vi "SERIAL_DecodeStreamResponse.vi"(8 "error in":errorcluster, 10 "Buffer":string, 11 "navX DevRef":T1={"SerialPortRef"={"DevStatus"={"status"=FALSE, "code"=0, "source"=""}, "Serial Port Name"=""}, "Board Information"={"WhoAmI (50 | 0x32)"=0, "Board Revision"=0, "Firmware Major Version"=0, "Firmware Minor Version"=0, "NAVX_BOARD_CAPABILITY"={"OMNIMOUNT"=FALSE, "YAW_RESET"=FALSE, "VEL_AND_DISP"=FALSE}, "NAVX_BOARD_YAW_AXIS"={"BOARD_YAW_AXIS_UP"=FALSE, "BOARD_YAW_AXIS"=0}}, "Status"={"Update Rate Hz"=0, "Accelerometer Full-Scale Range"=0, "Gyro Full-Scale Range"=0, "NAVX_OP_STATUS"=0, "NAVX_CAL_STATUS"=0, "NAVX_SELFTEST_STATUS"=0, "NAVX_SENSOR_STATUS"={"MOVING"=FALSE, "YAW_STABLE"=FALSE, "MAG_DISTURBANCE"=FALSE, "ALTITUDE_VALID"=FALSE, "SEALEVEL_PRESS_SET"=FALSE, "FUSED_HEADING_VALID"=FALSE}}, "Offsets"={"Yaw"=0.0, "Quat W"=0.0, "Quat X"=0.0, "Quat Y"=0.0, "Quat Z"=0.0}, "Update Rate (4Hz-60Hz)"=50, "Nav6Mode (YPR)"=enum."YPR", "refnum name"="", "error"={"status"=FALSE, "code"=0, "source"=""}, "Loop VI Refnum"=refnum} {"Status"."NAVX_OP_STATUS" items=["INITIALIZING", "SELFTEST_IN_PROGRESS", "ERROR", "IMU_AUTOCAL_IN_PROGRESS", "NORMAL"]; "Status"."NAVX_CAL_STATUS" items=["IMU_CAL_STATE_MASK"=3, "IMU_CAL_INPROGRESS"=0, "IMU_CAL_ACCUMULATE"=1, "IMU_CAL_COMPLETE"=2, "MAG_CAL_COMPLETE"=4, "BARO_CAL_COMPLETE"=8]}) -> (0 "error out":errorcluster, 2 "Valid":bool, 3 "navX DevRef":T1={"SerialPortRef"={"DevStatus"={"status"=FALSE, "code"=0, "source"=""}, "Serial Port Name"=""}, "Board Information"={"WhoAmI (50 | 0x32)"=0, "Board Revision"=0, "Firmware Major Version"=0, "Firmware Minor Version"=0, "NAVX_BOARD_CAPABILITY"={"OMNIMOUNT"=FALSE, "YAW_RESET"=FALSE, "VEL_AND_DISP"=FALSE}, "NAVX_BOARD_YAW_AXIS"={"BOARD_YAW_AXIS_UP"=FALSE, "BOARD_YAW_AXIS"=0}}, "Status"={"Update Rate Hz"=0, "Accelerometer Full-Scale Range"=0, "Gyro Full-Scale Range"=0, "NAVX_OP_STATUS"=0, "NAVX_CAL_STATUS"=0, "NAVX_SELFTEST_STATUS"=0, "NAVX_SENSOR_STATUS"={"MOVING"=FALSE, "YAW_STABLE"=FALSE, "MAG_DISTURBANCE"=FALSE, "ALTITUDE_VALID"=FALSE, "SEALEVEL_PRESS_SET"=FALSE, "FUSED_HEADING_VALID"=FALSE}}, "Offsets"={"Yaw"=0.0, "Quat W"=0.0, "Quat X"=0.0, "Quat Y"=0.0, "Quat Z"=0.0}, "Update Rate (4Hz-60Hz)"=50, "Nav6Mode (YPR)"=enum."YPR", "refnum name"="", "error"={"status"=FALSE, "code"=0, "source"=""}, "Loop VI Refnum"=refnum} {"Status"."NAVX_OP_STATUS" items=["INITIALIZING", "SELFTEST_IN_PROGRESS", "ERROR", "IMU_AUTOCAL_IN_PROGRESS", "NORMAL"]; "Status"."NAVX_CAL_STATUS" items=["IMU_CAL_STATE_MASK"=3, "IMU_CAL_INPROGRESS"=0, "IMU_CAL_ACCUMULATE"=1, "IMU_CAL_COMPLETE"=2, "MAG_CAL_COMPLETE"=4, "BARO_CAL_COMPLETE"=8]})   [LabVIEW 2014, in "navX-MXP IMU.lvlib"]
uses:
  navX-MXP IMU.lvlib
  navX Serial DevRef.ctl
  <vilib>/Rock Robotics/WPI/SerialPort/WPI_SerialPortRef.ctl
  COMMON/TypeDefs/Data TypeDefs/navX Board Information.ctl
  COMMON/TypeDefs/Value TypeDefs/navX NAVX_BOARD_CAPABILITY.ctl
  COMMON/TypeDefs/Value TypeDefs/navX NAVX_BOARD_YAW_AXIS.ctl
  COMMON/TypeDefs/Data TypeDefs/navX Status Data.ctl
  COMMON/TypeDefs/Value TypeDefs/navX NAVX_OP_STATUS.ctl
  COMMON/TypeDefs/Value TypeDefs/navX NAVX_CAL_STATUS.ctl
  COMMON/TypeDefs/Value TypeDefs/navX NAVX_SENSOR_STATUS.ctl
  TypeDefs/navX Serial Mode.ctl
  COMMON/TypeDefs/Data TypeDefs/navX Offsets Data.ctl
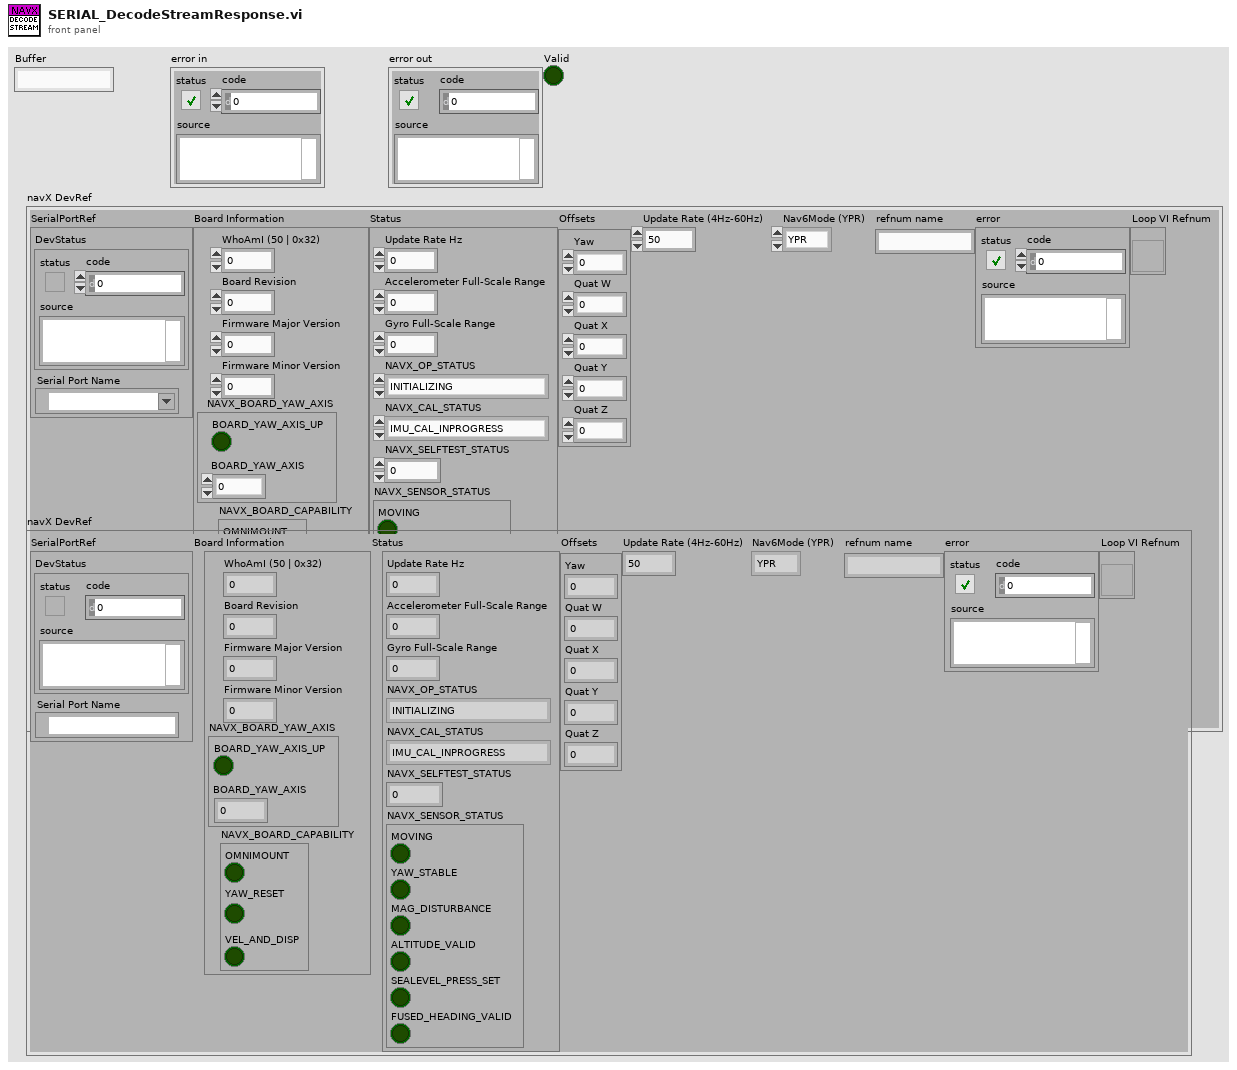
[diagram p1: front panel]
types:
  T1 = typedef "navX-MXP IMU.lvlib/navX Serial DevRef.ctl" = cluster{"SerialPortRef":T2, "Board Information":T3, "Status":T6, "Offsets":cluster{"Yaw":dbl, "Quat W":dbl, "Quat X":dbl, "Quat Y":dbl, "Quat Z":dbl}, "Update Rate (4Hz-60Hz)":u8, "Nav6Mode (YPR)":T10, "refnum name":string, "error":errorcluster, "Loop VI Refnum":refnum<vi>}
  T2 = typedef "WPI_SerialPortRef.ctl" = cluster{"DevStatus":errorcluster, "Serial Port Name":refnum<visa-resource-name>}
  T3 = typedef "navX-MXP IMU.lvlib/navX Board Information.ctl" = cluster{"WhoAmI (50 | 0x32)":u8, "Board Revision":u8, "Firmware Major Version":u8, "Firmware Minor Version":u8, "NAVX_BOARD_CAPABILITY":T4, "NAVX_BOARD_YAW_AXIS":T5}
  T4 = typedef "navX-MXP IMU.lvlib/navX NAVX_BOARD_CAPABILITY.ctl" = cluster{"OMNIMOUNT":bool, "YAW_RESET":bool, "VEL_AND_DISP":bool}
  T5 = typedef "navX-MXP IMU.lvlib/navX NAVX_BOARD_YAW_AXIS.ctl" = cluster{"BOARD_YAW_AXIS_UP":bool, "BOARD_YAW_AXIS":u8}
  T6 = typedef "navX-MXP IMU.lvlib/navX Status Data.ctl" = cluster{"Update Rate Hz":u8, "Accelerometer Full-Scale Range":u8, "Gyro Full-Scale Range":u16, "NAVX_OP_STATUS":T7, "NAVX_CAL_STATUS":T8, "NAVX_SELFTEST_STATUS":u8, "NAVX_SENSOR_STATUS":T9}
  T7 = typedef "navX-MXP IMU.lvlib/navX NAVX_OP_STATUS.ctl" = u8
  T8 = typedef "navX-MXP IMU.lvlib/navX NAVX_CAL_STATUS.ctl" = u8
  T9 = typedef "navX-MXP IMU.lvlib/navX NAVX_SENSOR_STATUS.ctl" = cluster{"MOVING":bool, "YAW_STABLE":bool, "MAG_DISTURBANCE":bool, "ALTITUDE_VALID":bool, "SEALEVEL_PRESS_SET":bool, "FUSED_HEADING_VALID":bool}
  T10 = typedef "navX-MXP IMU.lvlib/navX Serial Mode.ctl" = enum16{"YPR", "Gyro", "Quaternion"}
  T11 = typedef "navX-MXP IMU.lvlib/navX Offsets Data.ctl" = cluster{"Yaw":dbl, "Quat W":dbl, "Quat X":dbl, "Quat Y":dbl, "Quat Z":dbl}
  T12 = cluster{"Gyroscope Full Scale Range":u32, "Accelerometer Full Scale Range":u32, "Update Rate":u32, "Calibrated Yaw Offset":dbl, "Calibrated Quaternion W Offset ":u32, "Calibrated Quaternion X Offset":u32, "Calibrated Quaternion Y Offset":u32, "Calibrated Quaternion Z Offset":u32, "Flags":u32}
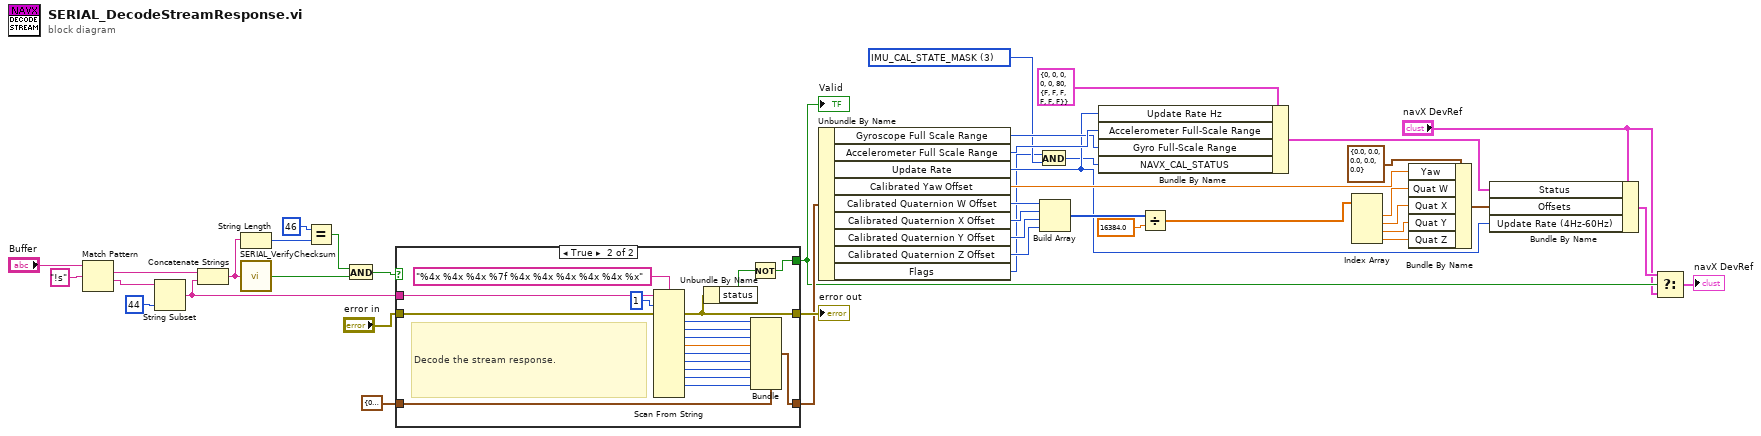
[diagram p0: block diagram]
diagram:
  w7 = T8 3 items=["IMU_CAL_STATE_MASK"=3, "IMU_CAL_INPROGRESS"=0, "IMU_CAL_ACCUMULATE"=1, "IMU_CAL_COMPLETE"=2, "MAG_CAL_COMPLETE"=4, "BARO_CAL_COMPLETE"=8] ("NAVX_CAL_STATUS")
  n1 = Match Pattern(string="Buffer", regular expression="!s") -> (match substring=w38:string, after substring=w40:string)  [unwired: 1 in, 2 out]
  n2 = String Subset(string=w40, length (rest)=44 ("length (rest)")) -> (substring=w28:string)  [unwired: 1 in]
  n3 = Concatenate Strings(w38, w28) -> (w29:string)
  n4 = String Length(string=w29) -> (length=w34:i32)
  n5 = call "SERIAL_VerifyChecksum.vi"("Content"=w29) -> ("Valid Checksum"=w37:bool)
  n6 = Equal?(x=46, y=w34) -> (x = y?=w32:bool)
  n7 = And(x=w32, y=w37) -> (x .and. y?=w36:bool)
  n8 = case shown="True" w36 {
    selector: w36 -> [w43 _]
    tunnel: [w44 w48] -> w35
    tunnel: w28 -> [_ w63]
    tunnel: [w45 w52] -> w27
    tunnel: T12 {"Gyroscope Full Scale Range"=0, "Accelerometer Full Scale Range"=0, "Update Rate"=0, "Calibrated Yaw Offset"=0.0, "Calibrated Quaternion W Offset "=0, "Calibrated Quaternion X Offset"=0, "Calibrated Quaternion Y Offset"=0, "Calibrated Quaternion Z Offset"=0, "Flags"=0} -> [w45 w51]
    tunnel: "error in" -> [w44 w50]
    tunnel: [w43 w46] -> w4
    frame False {
    }
    frame True {
      # "Decode the stream response."
      n9 = Scan From String(format string="%4x %4x %4x %7f %4x %4x %4x %4x %4x %x", input string=w63, initial scan location=u32 1, error in=w50) -> (error out=w48:errorcluster, output 1=w61:u32, output 2=w60:u32, output 3=w59:u32, output 4=w58:dbl, output 5=w57:u32, output 6=w56:u32, output 7=w55:u32, output 8=w54:u32, output 9=w53:u32)  [unwired: 11 in, 2 out]
      n10 = Unbundle By Name(w48) -> ("status"=w47:bool)
      n11 = Not(x=w47) -> (.not. x?=w46:bool)
      n12 = Bundle(cluster=w51, "Gyroscope Full Scale Range"=w61, "Accelerometer Full Scale Range"=w60, "Update Rate"=w59, "Calibrated Yaw Offset"=w58, "Calibrated Quaternion W Offset"=w57, "Calibrated Quaternion X Offset"=w56, "Calibrated Quaternion Y Offset"=w55, "Calibrated Quaternion Z Offset"=w54, "Flags"=w53) -> (w52:T12)
    }
  }
  "error out" <- w35
  "Valid" <- w4
  n13 = Unbundle By Name(w27) -> ("Gyroscope Full Scale Range"=w24:u32, "Accelerometer Full Scale Range"=w25:u32, "Update Rate"=w8:u32, "Calibrated Yaw Offset"=w23:dbl, "Calibrated Quaternion W Offset"=w22:u32, "Calibrated Quaternion X Offset"=w19:u32, "Calibrated Quaternion Y Offset"=w20:u32, "Calibrated Quaternion Z Offset"=w21:u32, "Flags"=w6:u32)
  n14 = And(x=w6, y=w7) -> (x .and. y?=w5:u32)
  n15 = Build Array(w22, w19, w20, w21) -> (w17:u32[])
  n16 = Bundle By Name(cluster=T6 {"Update Rate Hz"=0, "Accelerometer Full-Scale Range"=0, "Gyro Full-Scale Range"=0, "NAVX_OP_STATUS"=0, "NAVX_CAL_STATUS"=0, "NAVX_SELFTEST_STATUS"=80, "NAVX_SENSOR_STATUS"={"MOVING"=FALSE, "YAW_STABLE"=FALSE, "MAG_DISTURBANCE"=FALSE, "ALTITUDE_VALID"=FALSE, "SEALEVEL_PRESS_SET"=FALSE, "FUSED_HEADING_VALID"=FALSE}} ("Status"), "Update Rate Hz"=w8, "Accelerometer Full-Scale Range"=w25, "Gyro Full-Scale Range"=w24, "NAVX_CAL_STATUS"=w5) -> (w11:T6)
  n17 = Divide(x=w17, y=16384.0) -> (x/y=w16:dbl[])
  n18 = Index Array(array=w16) -> (element #1=w15:dbl, element #2=w14:dbl, element #3=w13:dbl, element #4=w12:dbl)  [unwired: 4 in]
  n19 = Bundle By Name(cluster=T11 {"Yaw"=0.0, "Quat W"=0.0, "Quat X"=0.0, "Quat Y"=0.0, "Quat Z"=0.0} ("Offsets"), "Yaw"=w23, "Quat W"=w15, "Quat X"=w14, "Quat Y"=w13, "Quat Z"=w12) -> (w9:T11)
  n20 = Bundle By Name(cluster="navX DevRef", "Status"=w11, "Offsets"=w9, "Update Rate (4Hz-60Hz)"=w8) -> (w3:T1)
  n21 = Select(t=w3, s=w4, f="navX DevRef") -> (s? t:f=→"navX DevRef":T1)
